vi "CRYAdd Steps Help.vi"(7 "Option":string, 8 "Coords":T1, 9 "Help":refnum<vi>, 10 "Help?":bool, 11 "AddSteps":refnum<vi>) -> ()   [LabVIEW 2013]
uses:
  <vilib>/Utility/miscctls.llb/LVPoint32TypeDef.ctl
  CRYProject/CRYProject Editor Global.vi
  CRYMainGlobal.vi
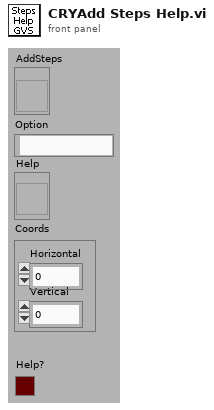
[diagram p1: front panel]
types:
  T1 = typedef "LVPoint32TypeDef.ctl" = cluster{"Horizontal":i32, "Vertical":i32}
  T2 = cluster{"Content":string, "Name":string, "Level":u32, "Category":string}[]
  T3 = cluster{"Content":string, "Name":string, "Level":u32, "Category":string}
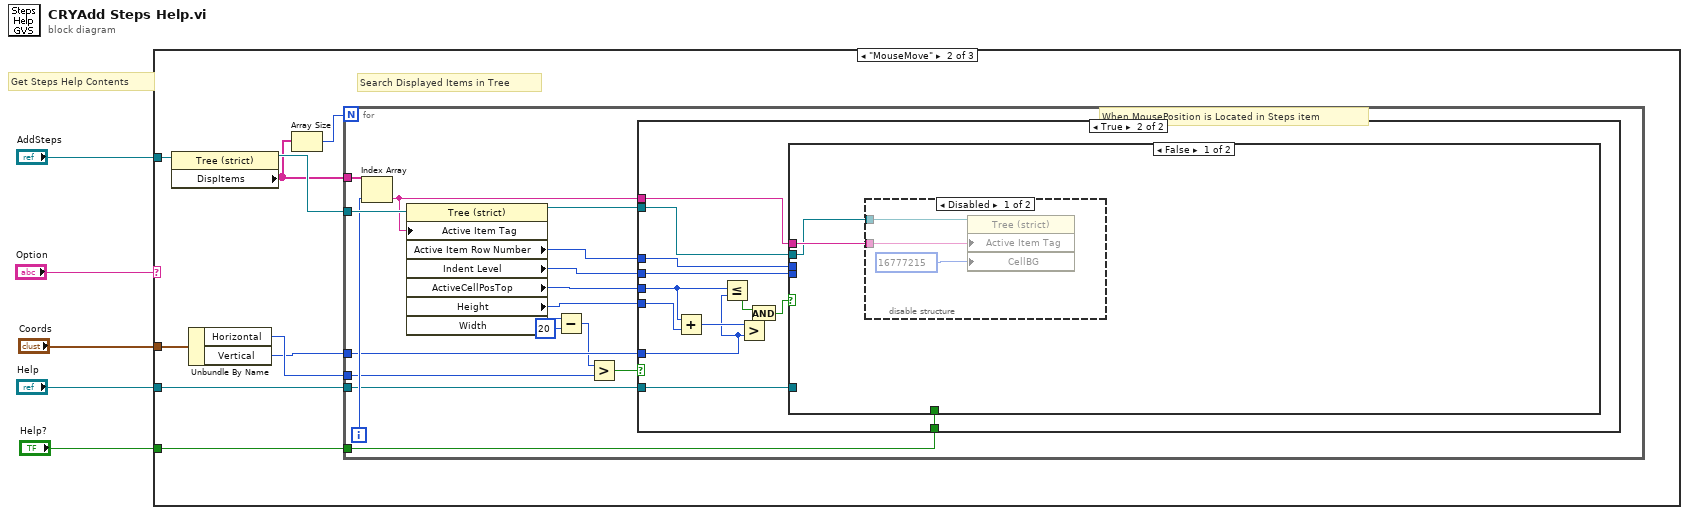
[diagram p0: block diagram]
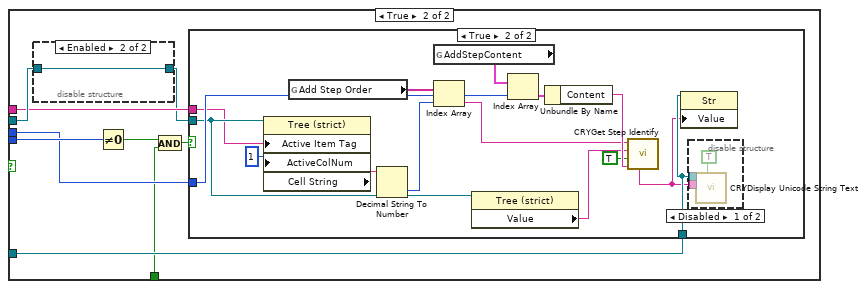
[diagram p5: hidden frame]
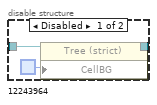
[diagram p6: hidden frame]
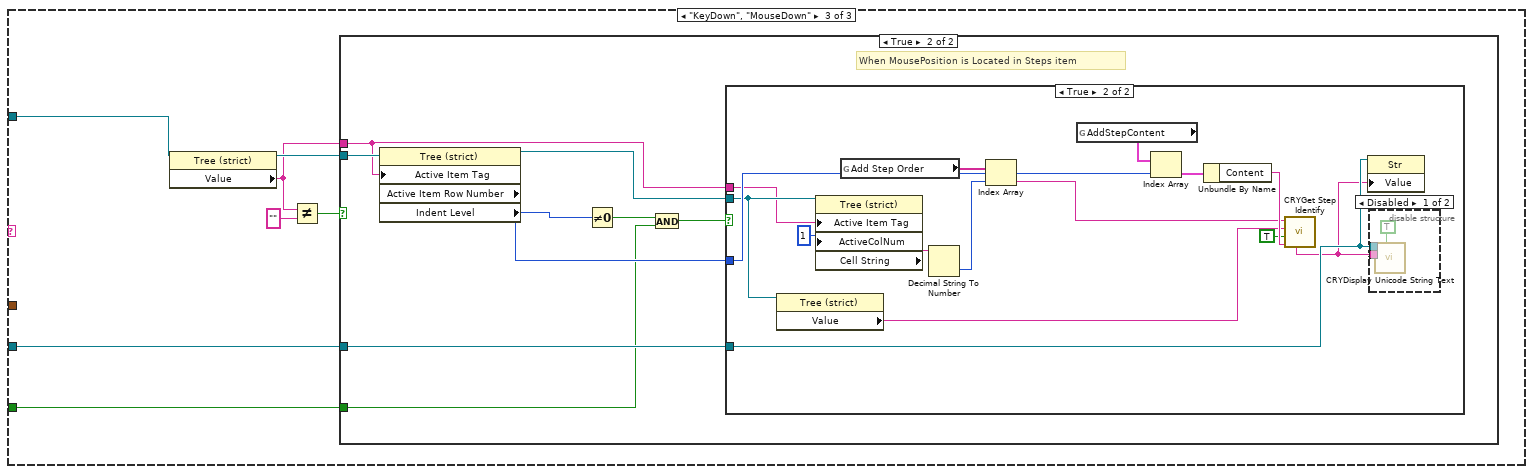
[diagram p9: hidden frame]
diagram:
  # "Get Steps Help Contents"
  n1 = case shown="\"MouseMove\"" "Option" {
    tunnel: "AddSteps" -> [_ w8 w84]
    tunnel: "Help" -> [_ w14 w86]
    tunnel: "Help?" -> [_ w13 w85]
    tunnel: "Coords" -> [_ w11 _]
    frame Default {
    }
    frame "MouseMove" {
      # "Search Displayed Items in Tree"
      n2 = property class="Tree (strict)"(reference=w8) -> (reference out=w7:refnum<vi>, "DispItems"=w6:string[])  [unwired: 1 in, 1 out]
      n3 = Unbundle By Name(w11) -> ("Horizontal"=w10:i32, "Vertical"=w9:i32)
      n4 = Array Size(array=w6) -> (size(s)=w12:i32)
      n5 = for {
        N: w12 -> [_]
        tunnel: w7 -> [w31]
        tunnel: w9 -> [w25]
        tunnel: w6 -> [w29]
        tunnel: w14 -> [w24]
        tunnel: w10 -> [w18]
        tunnel: w13 -> [w15]
        i -> [w30]
        # "When MousePosition is Located in Steps item"
        n6 = Index Array(array=w29, index=w30) -> (element=w28:string)
        n7 = property class="Tree (strict)"(reference=w31, "Active Item Tag"=w28) -> (reference out=w21:refnum<vi>, "Active Item Row Number"=w22:i32, "Indent Level"=w23:i32, "ActiveCellPosTop"=w27:i32, "Height"=w26:i32, "Width"=w20:i32)  [unwired: 1 in, 1 out]
        n8 = Subtract(x=w20, y=20) -> (x-y=w19:i32)
        n9 = Greater?(x=w19, y=w18) -> (0:w17:bool)
        n10 = case shown="True" w17 {
          tunnel: w28 -> [_ w41]
          tunnel: w27 -> [_ w40]
          tunnel: w26 -> [_ w38]
          tunnel: w25 -> [_ w37]
          tunnel: w24 -> [_ w36]
          tunnel: w23 -> [_ w35]
          tunnel: w22 -> [_ w34]
          tunnel: w21 -> [_ w33]
          tunnel: w15 -> [_ w32]
          frame False {
          }
          frame True {
            n11 = Add(x=w40, y=w38) -> (x+y=w39:i32)
            n12 = Less Or Equal?(x=w40, y=w37) -> (x <= y?=w43:bool)
            n13 = Greater?(x=w39, y=w37) -> (0:w44:bool)
            n14 = And(x=w43, y=w44) -> (x .and. y?=w42:bool)
            n15 = case shown="False" w42 {
              tunnel: w41 -> [w46 w57]
              tunnel: w33 -> [w45 w58]
              tunnel: w36 -> [_ w53]
              tunnel: w35 -> [_ w56]
              tunnel: w34 -> [_ w54]
              tunnel: w32 -> [_ w51]
              frame False {
                n16 = disable-structure shown="Disabled" {
                  disable-tunnel: w46 -> [w49 _]
                  disable-tunnel: w45 -> [w47 _]
                  frame Disabled {
                    n17 = property class="Tree (strict)"(reference=w47, "Active Item Tag"=w49, "CellBG"=u32 16777215 ("Active Cell:Background Color")) -> ()  [unwired: 1 in, 2 out]
                  }
                  frame Enabled {
                  }
                }
              }
              frame True {
                n18 = disable-structure shown="Enabled" {
                  disable-tunnel: w58 -> [w61 w62]
                  disable-tunnel: [w60 w62] -> w55
                  frame Disabled {
                    n19 = property on="Property Node" class="Tree (strict)"(reference=w61, "CellBG"=u32 12243964) -> (reference out=w60:refnum<vi>)  [unwired: 1 in, 1 out]
                  }
                  frame Enabled {
                  }
                }
                n20 = Not Equal To 0?(x=w56) -> (x != 0?=w52:bool)
                n21 = And(x=w52, y=w51) -> (x .and. y?=w50:bool)
                n22 = case shown="True" w50 {
                  tunnel: w57 -> [_ w64]
                  tunnel: w54 -> [_ w77]
                  tunnel: w55 -> [_ w65]
                  tunnel: w53 -> [_ w71]
                  frame False {
                  }
                  frame True {
                    n23 = property class="Tree (strict)"(reference=w65, "Active Item Tag"=w64, "ActiveColNum"=1 ("Active Cell:Active Column Number")) -> ("Cell String"=w67:string)  [unwired: 1 in, 2 out]
                    n24 = global read "CRYMainGlobal.vi" "Add Step Order"() -> (w68:string[])
                    n25 = Decimal String To Number(string=w67) -> (number=w69:i32)  [unwired: 2 in, 1 out]
                    n26 = global read "CRYProject Editor Global.vi" "AddStepContent"() -> (w76:T2)
                    n27 = Index Array(array=w68, index=w69) -> (element=w63:string)
                    n28 = property class="Tree (strict)"(reference=w65) -> ("Value"=w72:string)  [unwired: 1 in, 2 out]
                    n29 = Index Array(array=w76, index=w77) -> (element=w75:T3)
                    n30 = Unbundle By Name(w75) -> ("Content"=w74:string)
                    n31 = call "CRYGet Step Identify.vi"("Unflatten Seq-step setup"=w74, "Help?"=TRUE, "Value"=w72, "Category Name In"=w63) -> ("Help String"=w70:string)  [unwired: 7 out]
                    n32 = property class="Str"(reference=w71, "Value"=w70) -> ()  [unwired: 1 in, 2 out]
                    n33 = disable-structure shown="Disabled" {
                      disable-tunnel: w71 -> [w79 _]
                      disable-tunnel: w70 -> [w78 _]
                      frame Disabled {
                        n34 = call "CRYDisplay Unicode String Text.vi"("Interpret as Unicode (T)"=TRUE, "String Value"=w78, "String Control Reference"=w79) -> ()  [unwired: 5 in, 2 out]
                      }
                      frame Enabled {
                      }
                    }
                  }
                }
              }
            }
          }
        }
      }
    }
    frame "KeyDown", "MouseDown" {
      n35 = property class="Tree (strict)"(reference=w84) -> (reference out=w87:refnum<vi>, "Value"=w83:string)  [unwired: 1 in, 1 out]
      n36 = Not Equal?(x=w83, y="") -> (x != y?=w82:bool)
      n37 = case shown="True" w82 {
        tunnel: w87 -> [_ w93]
        tunnel: w83 -> [_ w92]
        tunnel: w86 -> [_ w89]
        tunnel: w85 -> [_ w88]
        frame False {
        }
        frame True {
          # "When MousePosition is Located in Steps item"
          n38 = property class="Tree (strict)"(reference=w93, "Active Item Tag"=w92) -> (reference out=w96:refnum<vi>, "Active Item Row Number"=w91:i32, "Indent Level"=w90:i32)  [unwired: 1 in, 1 out]
          n39 = Not Equal To 0?(x=w90) -> (x != 0?=w94:bool)
          n40 = And(x=w94, y=w88) -> (x .and. y?=w95:bool)
          n41 = case shown="True" w95 {
            tunnel: w92 -> [_ w98]
            tunnel: w91 -> [_ w111]
            tunnel: w96 -> [_ w99]
            tunnel: w89 -> [_ w105]
            frame False {
            }
            frame True {
              n42 = property class="Tree (strict)"(reference=w99) -> ("Value"=w106:string)  [unwired: 1 in, 2 out]
              n43 = property class="Tree (strict)"(reference=w99, "Active Item Tag"=w98, "ActiveColNum"=1 ("Active Cell:Active Column Number")) -> ("Cell String"=w101:string)  [unwired: 1 in, 2 out]
              n44 = global read "CRYMainGlobal.vi" "Add Step Order"() -> (w102:string[])
              n45 = Decimal String To Number(string=w101) -> (number=w103:i32)  [unwired: 2 in, 1 out]
              n46 = Index Array(array=w102, index=w103) -> (element=w97:string)
              n47 = global read "CRYProject Editor Global.vi" "AddStepContent"() -> (w110:T2)
              n48 = Index Array(array=w110, index=w111) -> (element=w109:T3)
              n49 = Unbundle By Name(w109) -> ("Content"=w108:string)
              n50 = call "CRYGet Step Identify.vi"("Unflatten Seq-step setup"=w108, "Help?"=TRUE, "Value"=w106, "Category Name In"=w97) -> ("Help String"=w104:string)  [unwired: 7 out]
              n51 = property class="Str"(reference=w105, "Value"=w104) -> ()  [unwired: 1 in, 2 out]
              n52 = disable-structure shown="Disabled" {
                disable-tunnel: w104 -> [w114 _]
                disable-tunnel: w105 -> [w112 _]
                frame Disabled {
                  n53 = call "CRYDisplay Unicode String Text.vi"("Interpret as Unicode (T)"=TRUE, "String Value"=w114, "String Control Reference"=w112) -> ()  [unwired: 5 in, 2 out]
                }
                frame Enabled {
                }
              }
            }
          }
        }
      }
    }
  }
